vi "SwissSPAD 1 Convert Data Info to String.vi"(5 "File Path":path, 6 "Step Duration":dbl[unit] format="%#.3g", 7 "Laser Period":dbl[unit], 8 "error in (no error)":errorcluster, 9 "size":i64, 10 "# Frames":u32, 11 "Swiss SPAD 1 File Information":T1 {"# Frames" format="%0.0f"; "Scan Increment (step unit)" format="%0.0f"; "Scan Start (step unit)" format="%0.0f"; "# Readouts/Frame" format="%0.0f"; "Initial Micro Shift" format="%0.0f"; "Initial Macro Shift" format="%0.0f"; "# Repetitions" format="%0.0f"; "Pattern Length" format="%0.0f"; "Gate Pattern" format="%064b"; "Recharge Pattern" format="%064b"; "SPAD Off Pattern" format="%064b"}) -> (0 "Error Out":errorcluster, 3 "Data Description":string)   [LabVIEW 2021, in "SwissSPAD.lvlib"]
uses:
  SwissSPAD1 File Information.ctl
  SwissSPAD.lvlib
  Variant/Variant.lvlib
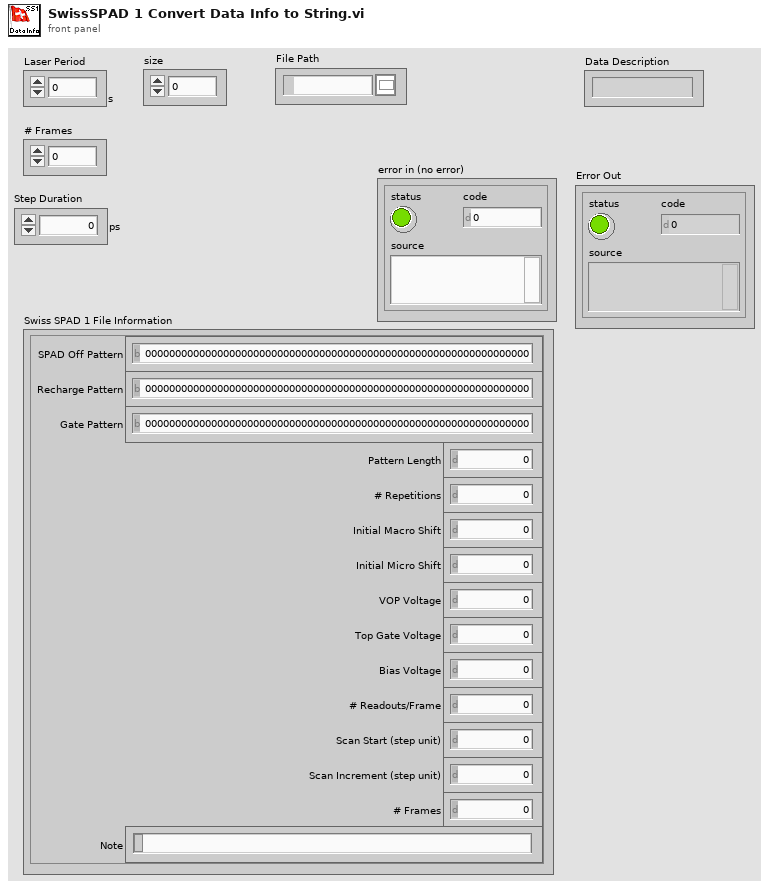
[diagram p1: front panel]
types:
  T1 = typedef "SwissSPAD.lvlib/SwissSPAD1 File Information.ctl" = cluster{"SPAD Off Pattern":u64, "Recharge Pattern":u64, "Gate Pattern":u64, "Pattern Length":u32, "# Repetitions":u32, "Initial Macro Shift":u32, "Initial Micro Shift":u32, "VOP Voltage":dbl, "Top Gate Voltage":dbl, "Bias Voltage":dbl, "# Readouts/Frame":u32, "Scan Start (step unit)":u32, "Scan Increment (step unit)":u32, "# Frames":u32, "Note":string}
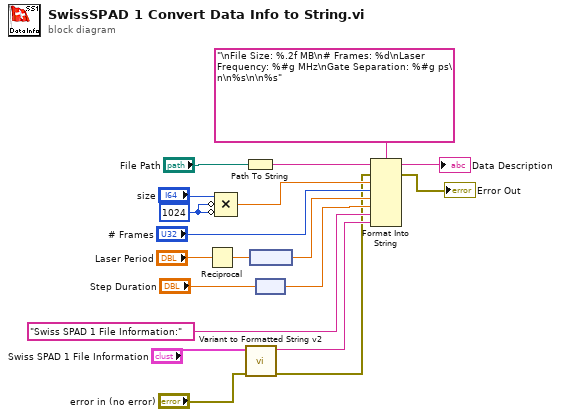
[diagram p0: block diagram]
diagram:
  w13 = i64 1024 ("y")
  n1 = Reciprocal(x="Laser Period") -> (1/x=w9:dbl[unit])
  n2 = Compound Arithmetic op=MULTIPLY("size", invert w13, invert w13) -> (w12:dbl)
  n3 = Path To String(path="File Path") -> (string=w16:string)
  n4 = call "Variant to Formatted String v2.vi"("error in (no error)"="error in (no error)", "Anything"="Swiss SPAD 1 File Information") -> ("error out"=w3:errorcluster, "String"=w4:string)  [unwired: 8 in]
  n5 = node(w9) -> (w8:dbl)
  n6 = node("Step Duration") -> (w6:dbl)
  n7 = Format Into String(format string="\nFile Size: %.2f MB\n# Frames: %d\nLaser Frequency: %#g MHz\nGate Separation: %#g ps\n\n%s\n\n%s", initial string=w16, error in=w3, w12, "# Frames", w8, w6, "Swiss SPAD 1 File Information:" ("Label"), w4) -> (resulting string=→"Data Description":string, error out=→"Error Out":errorcluster)
